vi "Main Page.vi"(8 "error in":errorcluster, 11 "Node Ptr":T1 format="%.0x") -> (0 "error out":errorcluster)   [LabVIEW 2017, in "Waveform-Processing-Custom-Device System Explorer.lvlib"]
uses:
  Waveform-Processing-Custom-Device System Explorer.lvlib
  <vilib>/NI Veristand/Custom Device API/Custom Device Item Ref.ctl
  Shared/Custom Device Settings.ctl
  Shared/Types/FG Action.ctl
  Types/UI Refs Ctl.ctl
  <vilib>/NI Veristand/Custom Device API/Custom Device API.lvlib
  Shared/Single Point/SinglePoint.lvlib
  Shared/Running Average/Running Average.lvlib
  Shared/Waveform-Processing-Custom-Device Shared.lvlib
  Shared/Min Single Point/Min_SP.lvlib
  Shared/Max Single Point/Max_SP.lvlib
panel:
  in  "RMS":bool
  in  "Max":bool
  in  "Min":bool
  out "Number of Channels":u32 caption="# Ch's"
  in  "Refresh Waveform List":bool
  out "Revision":string
  in  "Header 2":cluster{"Section Name":string}={"Section Name"="Custom Device Item Settings"}
  out "Task Rate":dbl caption="Hz"
  in  "Buffer Length":dbl=1.0 caption="Sec" min=1.0 format="%#_6f"
  out "Buffer Length":u32 caption="Samples"
  in  "Description":string
  in  "Remove Channel":bool
  in  "Add Channel":bool
  in  "Selected Waveforms":i32[](listbox)
  in  "Waveform Task":u16(ring) items=["Waveform1"=11, "Waveform2"=15]
  in  "Available Waveforms":i32[](listbox)
  in  "Single-point":bool
  in  "Header":cluster{"Section Name":string}={"Section Name"="Custom Device Item Settings"}
  in  "Name":string
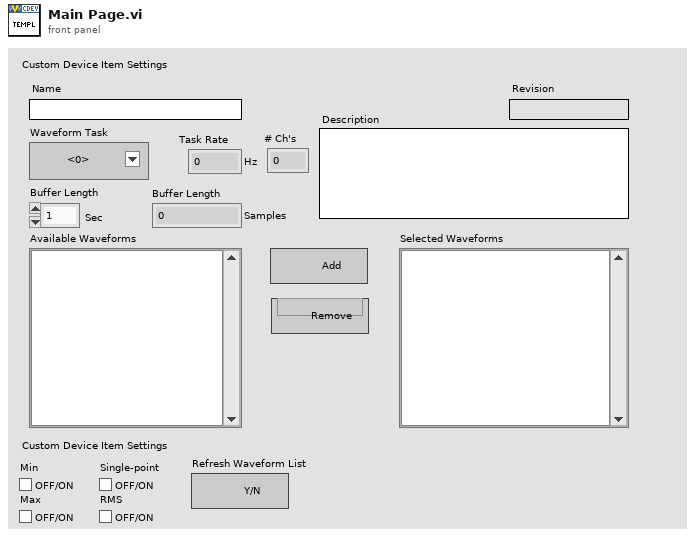
[diagram p1: front panel]
types:
  T1 = typedef "Custom Device API.lvlib/Custom Device Item Ref.ctl" = u64
  T2 = typedef "Waveform-Processing-Custom-Device Shared.lvlib/Custom Device Settings.ctl" = cluster{"CD Task Dependency":T1, "CD Task Dependency Ref":T1, "CD Task Available Wfms":string[], "CD Task Selected Wfms":string[], "Buffer Length (samples)":u32, "Min Enabled":bool, "Max Enabled ":bool, "SP Enabled":bool, "RMS Enabled":bool, "Buffer Length (s)":dbl, "Task Rate":dbl, "Number of DAQ Chanels":u32}
  T3 = typedef "Waveform-Processing-Custom-Device Shared.lvlib/UI Refs Ctl.ctl" = cluster{"Waveform Task":refnum<vi>, "Selected Waveforms":refnum<vi>, "Available Waveforms":refnum<vi>, "Number of Channels":refnum<vi>, "Wfm Task Rate (Hz)":refnum<vi>, "Buffer Length (s)":refnum<vi>, "Buffer Length (samples)":refnum<vi>, "Add Channel":refnum<vi>, "Remove Channel":refnum<vi>, "Min":refnum<vi>, "Max":refnum<vi>, "SP":refnum<vi>, "RMS":refnum<vi>}
  T4 = typedef "Waveform-Processing-Custom-Device Shared.lvlib/FG Action.ctl" = enum8{"GET", "SET"}
  T5 = typedef "Custom Device API.lvlib/Custom Device Item Info.ctl" = cluster{"Name":string, "Is Channel":bool, "GUID":string, "Is Waveform":bool}
  T6 = enum8{"Enabled", "Disabled", "Disabled and Grayed Out"}
  T7 = typedef "Custom Device API.lvlib/Custom Device Commands.ctl" = enum16{"Default", "Item renamed", "Shutdown", "Dynamic button pressed"}
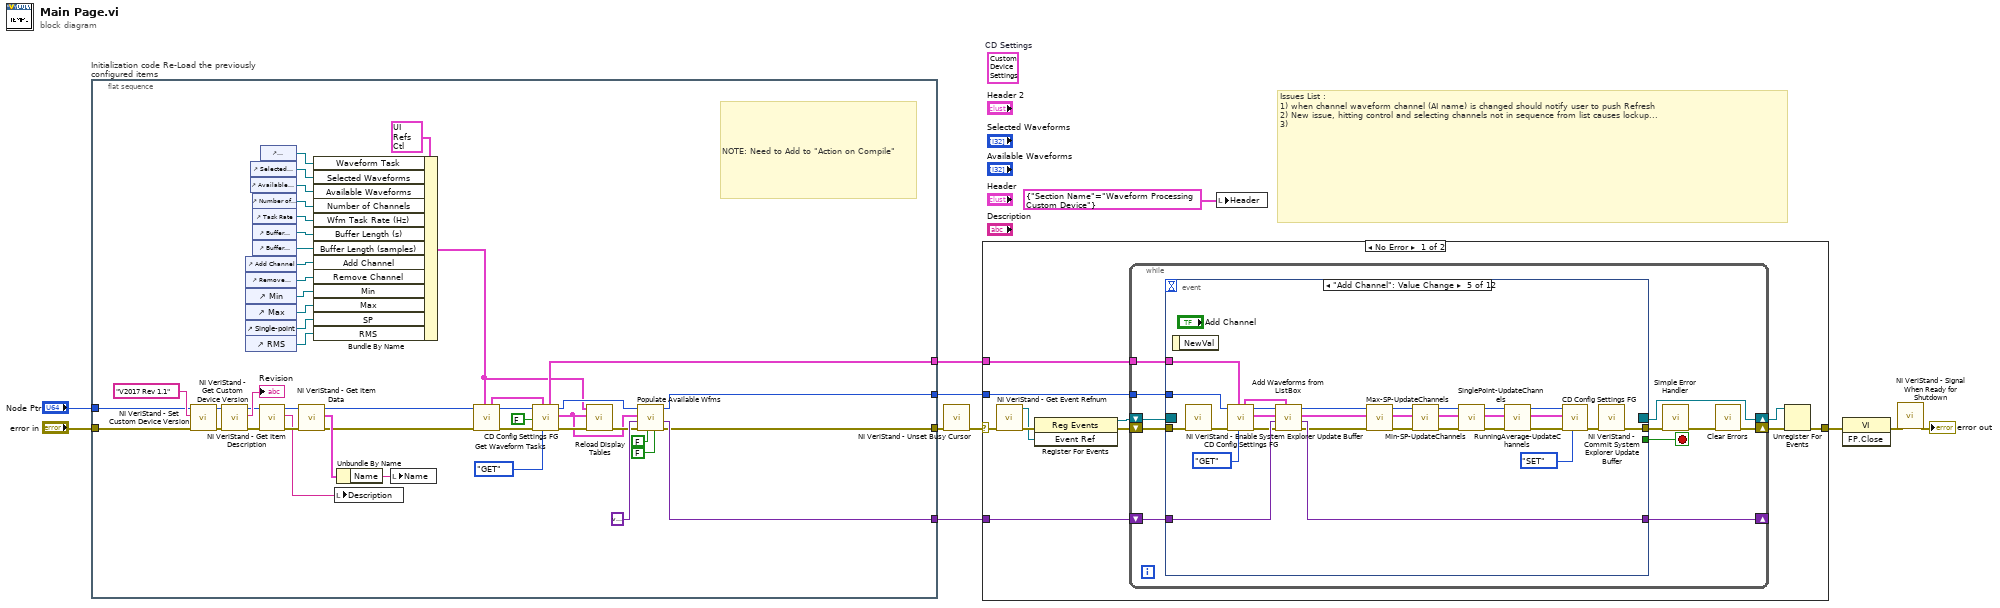
[diagram p0: block diagram]
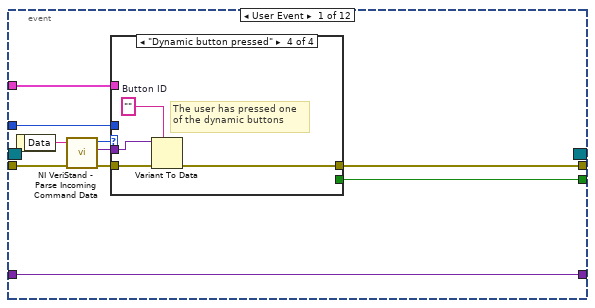
[diagram p2: hidden frame]
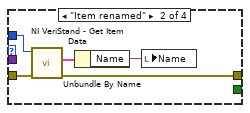
[diagram p4: hidden frame]
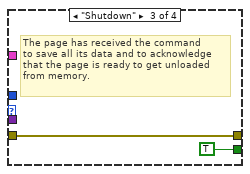
[diagram p5: hidden frame]
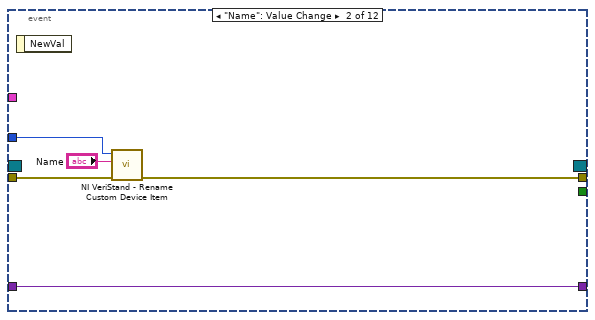
[diagram p6: hidden frame]
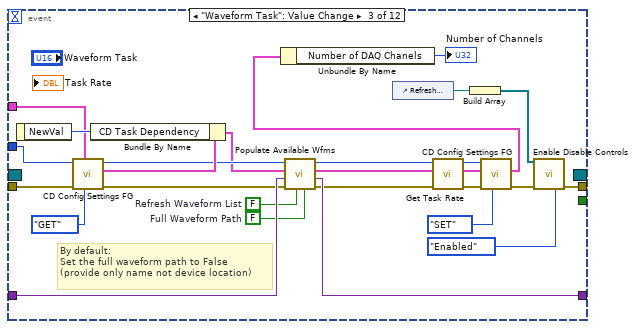
[diagram p7: hidden frame]
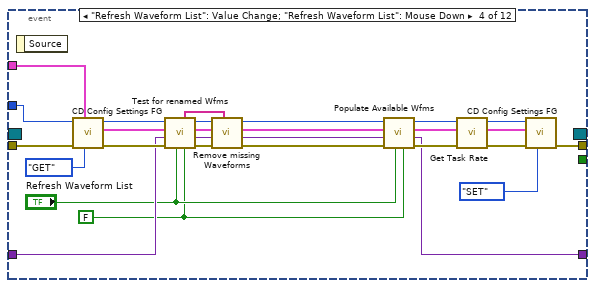
[diagram p8: hidden frame]
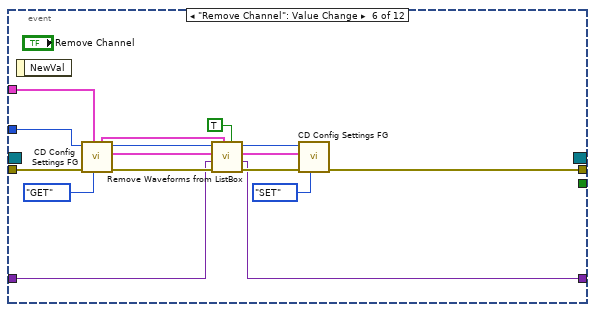
[diagram p9: hidden frame]
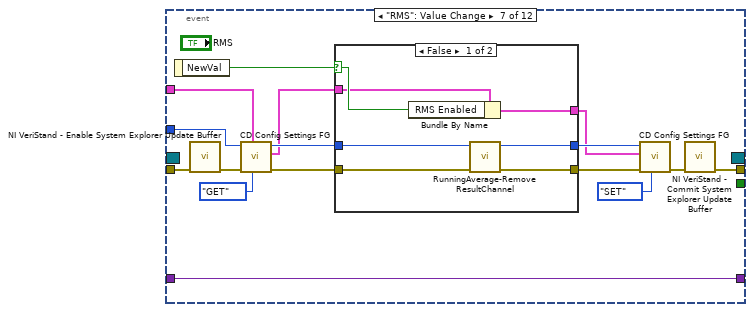
[diagram p10: hidden frame]
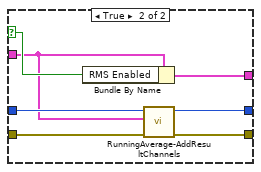
[diagram p11: hidden frame]
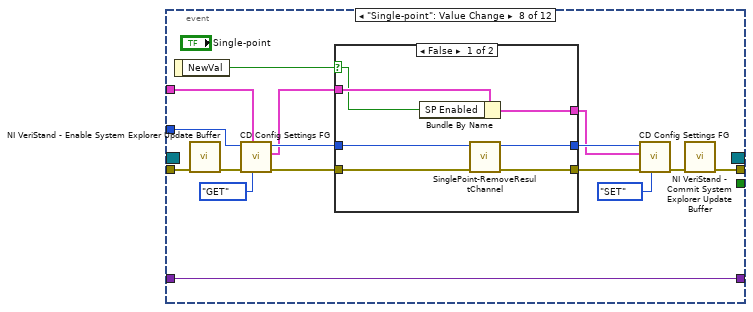
[diagram p12: hidden frame]
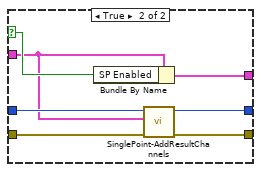
[diagram p13: hidden frame]
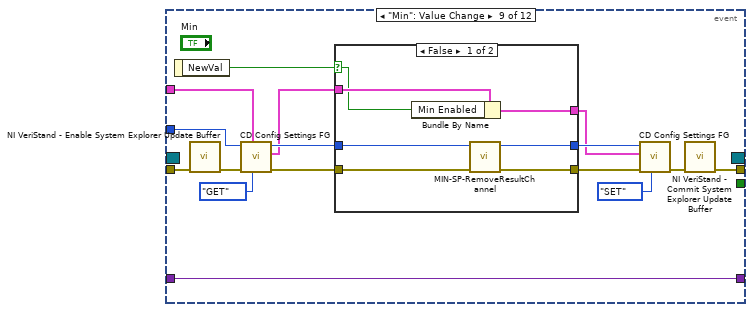
[diagram p14: hidden frame]
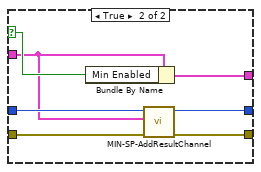
[diagram p15: hidden frame]
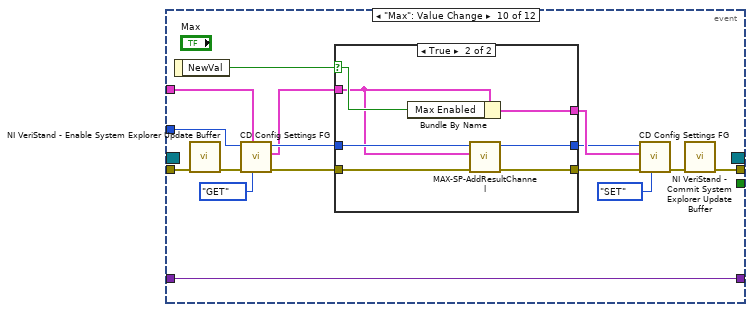
[diagram p16: hidden frame]
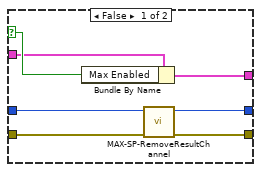
[diagram p17: hidden frame]
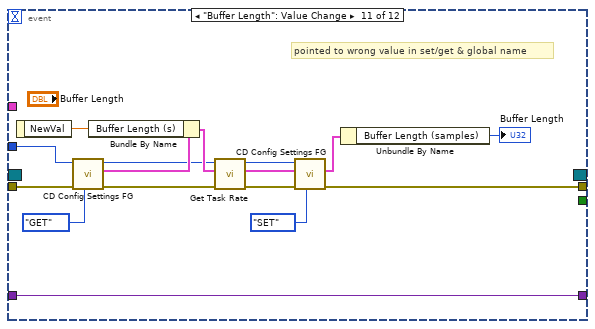
[diagram p18: hidden frame]
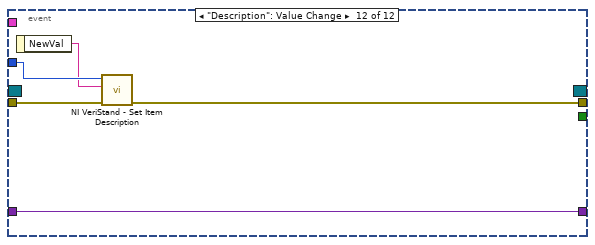
[diagram p19: hidden frame]
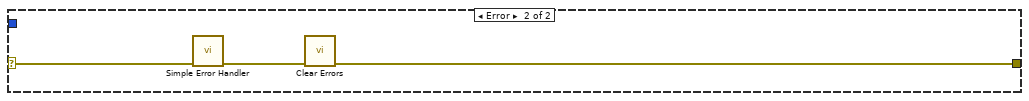
[diagram p20: hidden frame]
diagram:
  (unwired) T2 {"CD Task Dependency"=18446744073709551615, "CD Task Dependency Ref"=18446744073709551615, "CD Task Available Wfms"=[], "CD Task Selected Wfms"=[], "Buffer Length (samples)"=0, "Min Enabled"=FALSE, "Max Enabled "=FALSE, "SP Enabled"=FALSE, "RMS Enabled"=FALSE, "Buffer Length (s)"=0.0, "Task Rate"=0.0, "Number of DAQ Chanels"=0}  # CD Settings
  # "Issues List : \n1) when channel waveform channel (AI name) is changed should notify user to push Refresh\n2) New issue, hitting control and selecting channels not in sequence from list causes lockup...\n3)"
  n1 = flat-sequence "Initialization code Re-Load the previously configured items" {
    tunnel: [w51] -> w4
    tunnel: [w35] -> w7
    tunnel: [w47] -> w6
    tunnel: [w17] -> w5
    tunnel: "error in" -> [w30]
    tunnel: "Node Ptr" -> [w40]
    frame #0 {
      # "NOTE: Need to Add to \"Action on Compile\""
      n2 = call <vilib>:"NI VeriStand - Set Custom Device Version.vi"("error in (no error)"=w30, "Value"="V2017 Rev 1.1", "Device Ref in"=w40) -> ("error out"=w44:errorcluster, "Device Ref out"=w45:T1)  [unwired: 7 in]
      n3 = call <vilib>:"NI VeriStand - Get Custom Device Version.vi"("error in (no error)"=w44, "Device Ref in"=w45) -> ("error out"=w42:errorcluster, "Value"=→"Revision":string, "Device Ref out"=w41:T1)  [unwired: 7 in]
      n4 = control-ref of="Add Channel"() -> (w23:refnum<vi>)
      n5 = control-ref of="Remove Channel"() -> (w22:refnum<vi>)
      n6 = control-ref of="Min"() -> (w13:refnum<vi>)
      n7 = control-ref of="Max"() -> (w21:refnum<vi>)
      n8 = control-ref of="Single-point"() -> (w20:refnum<vi>)
      n9 = control-ref of="RMS"() -> (w19:refnum<vi>)
      n10 = control-ref of="Selected Waveforms"() -> (w28:refnum<vi>)
      n11 = control-ref of="Available Waveforms"() -> (w27:refnum<vi>)
      n12 = control-ref of="Number of Channels"() -> (w26:refnum<vi>)
      n13 = control-ref of="Task Rate"() -> (w25:refnum<vi>)
      n14 = control-ref of="Buffer Length"() -> (w24:refnum<vi>)
      n15 = control-ref of="Buffer Length"() -> (w18:refnum<vi>)
      n16 = call <vilib>:"NI VeriStand - Get Item Description.vi"("error in (no error)"=w42, "Item Ref in"=w41) -> ("error out"=w56:errorcluster, "Description"=w53:string, "Item Ref out"=w57:T1)  [unwired: 7 out]
      n17 = control-ref of="Waveform Task"() -> (w29:refnum<vi>)
      n18 = call <vilib>:"NI VeriStand - Get Item Data.vi"("error in (no error)"=w56, "Item Ref in"=w57) -> ("error out"=w36:errorcluster, "Item Info"=w55:T5, "Item Ref out"=w14:T1)  [unwired: 7 out]
      n19 = Bundle By Name(cluster=T3 {"Waveform Task"=refnum, "Selected Waveforms"=refnum, "Available Waveforms"=refnum, "Number of Channels"=refnum, "Wfm Task Rate (Hz)"=refnum, "Buffer Length (s)"=refnum, "Buffer Length (samples)"=refnum, "Add Channel"=refnum, "Remove Channel"=refnum, "Min"=refnum, "Max"=refnum, "SP"=refnum, "RMS"=refnum} ("UI Refs"), "Waveform Task"=w29, "Selected Waveforms"=w28, "Available Waveforms"=w27, "Number of Channels"=w26, "Wfm Task Rate (Hz)"=w25, "Buffer Length (s)"=w24, "Buffer Length (samples)"=w18, "Add Channel"=w23, "Remove Channel"=w22, "Min"=w13, "Max"=w21, "SP"=w20, "RMS"=w19) -> (w16:T3)
      n20 = local write "Description"(w53) -> ()
      n21 = Unbundle By Name(w55) -> ("Name"=w54:string)
      n22 = local write "Name"(w54) -> ()
      n23 = call "Get Waveform Tasks.vi"("Custom Device ref in"=w14, "error in"=w36, "UI Refs in"=w16) -> ("UI Refs out"=w15:T3, "Custom Device ref out"=w48:T1, "error out"=w34:errorcluster)  [unwired: 5 in]
      n24 = call "CD Config Settings FG.vi"("Action"=FG_Action."GET", "UI Refs"=w15, "Error In"=w34, "Force"=FALSE, "Item Ref"=w48) -> ("Error Out"=w33:errorcluster, "CD Settings out"=w12:T2, "Item Ref out"=w39:T1, "UI Refs out"=w17:T3)  [unwired: 3 in]
      n25 = call "Reload Display Tables.vi"("Error In"=w33, "CD Settings In"=w12, "UI Refs In"=w16) -> ("Error Out"=w32:errorcluster)  [unwired: 8 in]
      n26 = call "Populate Available Wfms.vi"("Full Path info"=FALSE, "Refresh List"=FALSE, "Error In"=w32, "ListBox Variant"=variant, "CD Settings"=w12, "CustomDevice Ref"=w39) -> ("Error Out"=w35:errorcluster, "ListBox Variant"=w51:variant, "CustomDevice Ref"=w47:T1)  [unwired: 1 in, 2 out]
    }
  }
  n27 = call <vilib>:"NI VeriStand - Unset Busy Cursor.vi"("error in (no error)"=w7) -> ("error out"=w8:errorcluster)  [unwired: 10 out]
  n28 = case shown="No Error" w8 {
    selector: w8 -> [w61 w350]
    tunnel: [w65 w348] -> w11
    tunnel: w6 -> [w60 _]
    tunnel: w4 -> [w59 _]
    tunnel: w5 -> [w58 _]
    frame No Error {
      n29 = call <vilib>:"NI VeriStand - Get Event Refnum.vi"("error in (no error)"=w61) -> ("error out"=w68:errorcluster, "Event Ref"=w64:refnum<user-event>)  [unwired: 9 out]
      n30 = register-events(error in=w68, w64) -> (reference out=w62:refnum<event-registration>, error out=w63:errorcluster)  [unwired: 1 in]
      n31 = while {
        shift-right: [w75] -> w66
        shift-left: w63 -> [w72]
        shift-right: [w79] -> w67
        shift-left: w62 -> [w78]
        tunnel: w60 -> [w74]
        shift-right: [w70] -> _
        shift-left: w59 -> [w73]
        tunnel: w58 -> [w69]
        stop <- w77 stop-if-true
        n32 = event shown="[4] \"Add Channel\": Value Change" {
          selector: w78 -> [_ _ _ _ _ _ _ _ _ _ _ _]
          dyn-events: [_ _ _ _ _ _ _ _ _ _ _ _] -> w79
          timeout: _ -> [_ _ _ _ _ _ _ _ _ _ _ _]
          tunnel: w72 -> [w89 w106 w118 w161 w178 w203 w212 w238 w269 w299 w341 w347]
          tunnel: [w85 _ _ _ _ _ _ _ _ _ _ _] -> w77
          tunnel: [w84 w105 w116 w151 w174 w195 w207 w240 w271 w300 w331 w346] -> w71
          tunnel: w74 -> [w82 w103 w130 w160 w190 w206 w218 w247 w276 w310 w330 w345]
          tunnel: [w81 w102 w133 w137 w182 w192 w221 w251 w282 w312 w342 w343] -> w70
          tunnel: w73 -> [w81 w102 w132 w148 w185 w194 w221 w251 w282 w312 w342 w343]
          tunnel: w69 -> [w80 _ w121 w134 w181 w193 w215 w248 w274 w311 _ _]
          event User Event {
            n33 = event-data() -> ("Data"=w88:string)  [unwired: 1 out]
            n34 = call <vilib>:"NI VeriStand - Parse Incoming Command Data.vi"("error in (no error)"=w89, "Incoming data"=w88) -> ("error out"=w87:errorcluster, "Outgoing data"=w83:variant, "Action"=w86:T7)  [unwired: 7 out]
            n35 = case shown="\"Dynamic button pressed\"" w86 {
              tunnel: w87 -> [w90 w95 w96 w101]
              tunnel: [_ _ TRUE _] -> w85
              tunnel: [w90 w93 w96 w98] -> w84
              tunnel: w83 -> [_ _ _ w100]
              tunnel: w82 -> [_ w91 _ _]
              tunnel: w80 -> [_ _ _ _]
              frame "Default", Default {
              }
              frame "Item renamed" {
                n36 = call <vilib>:"NI VeriStand - Get Item Data.vi"("error in (no error)"=w95, "Item Ref in"=w91) -> ("error out"=w93:errorcluster, "Item Info"=w94:T5)  [unwired: 8 out]
                n37 = Unbundle By Name(w94) -> ("Name"=w92:string)
                n38 = local write "Name"(w92) -> ()
              }
              frame "Shutdown" {
                # "The page has received the command \nto save all its data and to acknowledge \nthat the page is ready to get unloaded \nfrom memory."
              }
              frame "Dynamic button pressed" {
                w99 = ""  # Button ID
                # "The user has pressed one \nof the dynamic buttons"
                n39 = Variant To Data(error in=w101, type=w99, Variant=w100) -> (error out=w98:errorcluster)  [unwired: 1 out]
              }
            }
          }
          event "Name": Value Change {
            n40 = event-data() -> ()  [unwired: 2 out]
            n41 = call <vilib>:"NI VeriStand - Rename Custom Device Item.vi"("error in (no error)"=w106, "New Name"="Name", "Item Ref in"=w103) -> ("error out"=w105:errorcluster)  [unwired: 1 in, 7 out]
          }
          event "Waveform Task": Value Change {
            w119 = FALSE  # Full Waveform Path
            w120 = FALSE  # Refresh Waveform List
            # "By default:\nSet the full waveform path to False \n(provide only name not device location)"
            n42 = event-data() -> ("NewVal"=w131:u16)  [unwired: 1 out]
            n43 = call "CD Config Settings FG.vi"("Action"=FG_Action."GET", "UI Refs"=w121, "Error In"=w118, "Item Ref"=w130) -> ("Error Out"=w126:errorcluster, "CD Settings out"=w129:T2, "Item Ref out"=w125:T1)  [unwired: 4 in, 1 out]
            n44 = Bundle By Name(cluster=w129, "CD Task Dependency"=w131) -> (w124:T2)
            n45 = call "Populate Available Wfms.vi"("Full Path info"=w119, "Refresh List"=w120, "Error In"=w126, "ListBox Variant"=w132, "CD Settings"=w124, "CustomDevice Ref"=w125) -> ("Error Out"=w112:errorcluster, "ListBox Variant"=w133:variant, "CD Settings out"=w110:T2, "CustomDevice Ref"=w111:T1)  [unwired: 1 in, 1 out]
            n46 = control-ref of="Refresh Waveform List"() -> (w114:refnum<vi>)
            n47 = call "Get Task Rate.vi"("error in"=w112, "CD Settings"=w110, "CustomDevice Ref"=w111) -> ("error out"=w122:errorcluster, "CD Settings out"=w109:T2, "CustomDevice Ref out"=w123:T1)  [unwired: 6 in]
            n48 = Build Array(w114) -> (w113:refnum<vi>[])
            n49 = call "CD Config Settings FG.vi"("Action"=FG_Action."SET", "Error In"=w122, "CD Settings in"=w109, "Item Ref"=w123) -> ("Error Out"=w117:errorcluster, "CD Settings out"=w108:T2)  [unwired: 4 in, 2 out]
            n50 = Unbundle By Name(w108) -> ("Number of DAQ Chanels"=→"Number of Channels":u32)
            n51 = call "Enable Disable Controls.vi"("Control Group 1"=w113, "Error In"=w117, "Control Group 1 Mode"=T6."Enabled" ("Disabled")) -> ("Error Out"=w116:errorcluster)  [unwired: 12 in]
          }
          event "Refresh Waveform List": Value Change; "Refresh Waveform List": Mouse Down {
            w135 = FALSE ("Full Waveform Path")
            n52 = event-data() -> ()  [unwired: 2 out]
            n53 = call "CD Config Settings FG.vi"("Action"=FG_Action."GET", "UI Refs"=w134, "Error In"=w161, "Item Ref"=w160) -> ("Error Out"=w150:errorcluster, "CD Settings out"=w147:T2, "Item Ref out"=w149:T1)  [unwired: 4 in, 1 out]
            n54 = call "Test for renamed Wfms.vi"("Full Path info"=w135, "Refresh List"="Refresh Waveform List", "Error In"=w150, "ListBox Variant"=w148, "CD Settings"=w147, "CustomDevice Ref"=w149) -> ("Error Out"=w142:errorcluster, "ListBox Variant"=w144:variant, "CD Settings out"=w139:T2, "CustomDevice Ref"=w145:T1, "Names to Remove"=w140:string[])  [unwired: 1 in]
            n55 = call "Remove missing Waveforms.vi"("Names to Remove"=w140, "Error In"=w142, "ListBox Variant In"=w144, "CD Settings in"=w139, "Item Ref In"=w145) -> ("Error Out"=w141:errorcluster, "ListBox Variant Out"=w143:variant, "CD Settings out"=w138:T2, "Item Ref Out"=w146:T1)  [unwired: 3 in]
            n56 = call "Populate Available Wfms.vi"("Full Path info"=w135, "Refresh List"="Refresh Waveform List", "Error In"=w141, "ListBox Variant"=w143, "CD Settings"=w138, "CustomDevice Ref"=w146) -> ("Error Out"=w157:errorcluster, "ListBox Variant"=w137:variant, "CD Settings out"=w156:T2, "CustomDevice Ref"=w155:T1)  [unwired: 1 in, 1 out]
            n57 = call "Get Task Rate.vi"("error in"=w157, "CD Settings"=w156, "CustomDevice Ref"=w155) -> ("error out"=w153:errorcluster, "CD Settings out"=w152:T2, "CustomDevice Ref out"=w154:T1)  [unwired: 6 in]
            n58 = call "CD Config Settings FG.vi"("Action"=FG_Action."SET", "Error In"=w153, "CD Settings in"=w152, "Item Ref"=w154) -> ("Error Out"=w151:errorcluster)  [unwired: 4 in, 3 out]
          }
          event "Add Channel": Value Change {
            n59 = event-data() -> ()  [unwired: 2 out]
            n60 = call <vilib>:"NI VeriStand - Enable System Explorer Update Buffer.vi"("error in (no error)"=w178) -> ("error out"=w177:errorcluster)  [unwired: 10 in]
            n61 = call "CD Config Settings FG.vi"("Action"=FG_Action."GET", "UI Refs"=w181, "Error In"=w177, "Item Ref"=w190) -> ("Error Out"=w184:errorcluster, "CD Settings out"=w187:T2, "Item Ref out"=w186:T1, "UI Refs out"=w183:T3)  [unwired: 4 in]
            n62 = call "Add Waveforms from ListBox.vi"("UI Refs"=w183, "error in"=w184, "Wfm Ref LUT"=w185, "CD Settings in"=w187, "Custom Device Ref in"=w186) -> ("error out"=w176:errorcluster, "Wfm Ref LUT out"=w182:variant, "CD Settings out"=w179:T2, "Custom Device Ref out"=w180:T1)  [unwired: 3 in]
            n63 = call "Max-SP-UpdateChannels.vi"("Error In"=w176, "CD Settings In"=w179, "Item Ref in"=w180) -> ("Error Out"=w172:errorcluster, "CD Settings Out"=w171:T2, "Item Ref Out"=w173:T1)  [unwired: 6 in]
            n64 = call "Min-SP-UpdateChannels.vi"("Error In"=w172, "CD Settings In"=w171, "Item Ref in"=w173) -> ("Error Out"=w168:errorcluster, "CD Settings Out"=w169:T2, "Item Ref Out"=w170:T1)  [unwired: 6 in]
            n65 = call "SinglePoint-UpdateChannels.vi"("Error in"=w168, "CD Settings In"=w169, "Custom Device ref in"=w170) -> ("Error out"=w163:errorcluster, "CD Settings Out"=w165:T2, "Custom Device ref out"=w167:T1)  [unwired: 6 in]
            n66 = call "RunningAverage-UpdateChannels.vi"("Error in"=w163, "CD Settings In"=w165, "Custom Device ref in"=w167) -> ("Error out"=w162:errorcluster, "CD Settings"=w164:T2, "Custom Device ref out"=w166:T1)  [unwired: 6 in]
            n67 = call "CD Config Settings FG.vi"("Action"=FG_Action."SET", "Error In"=w162, "CD Settings in"=w164, "Item Ref"=w166) -> ("Error Out"=w175:errorcluster)  [unwired: 4 in, 3 out]
            n68 = call <vilib>:"NI VeriStand - Commit System Explorer Update Buffer.vi"("error in (no error)"=w175) -> ("error out"=w174:errorcluster)  [unwired: 10 in]
          }
          event "Remove Channel": Value Change {
            n69 = event-data() -> ()  [unwired: 2 out]
            n70 = call "CD Config Settings FG.vi"("Action"=FG_Action."GET", "UI Refs"=w193, "Error In"=w203, "Item Ref"=w206) -> ("Error Out"=w202:errorcluster, "CD Settings out"=w200:T2, "Item Ref out"=w199:T1, "UI Refs out"=w198:T3)  [unwired: 4 in]
            n71 = call "Remove Waveforms from ListBox.vi"("Names List"=TRUE, "UI Refs"=w198, "error in"=w202, "Waveform Ref LUT"=w194, "CD Settings in"=w200, "Custom Device Ref in"=w199) -> ("error out"=w201:errorcluster, "Waveform Ref LUT out"=w192:variant, "CD Settings out"=w196:T2, "Custom Device Ref out"=w197:T1)  [unwired: 2 in]
            n72 = call "CD Config Settings FG.vi"("Action"=FG_Action."SET", "Error In"=w201, "CD Settings in"=w196, "Item Ref"=w197) -> ("Error Out"=w195:errorcluster)  [unwired: 4 in, 3 out]
          }
          event "RMS": Value Change {
            n73 = event-data() -> ("NewVal"=w222:bool)  [unwired: 1 out]
            n74 = call <vilib>:"NI VeriStand - Enable System Explorer Update Buffer.vi"("error in (no error)"=w212) -> ("error out"=w211:errorcluster)  [unwired: 10 in]
            n75 = call "CD Config Settings FG.vi"("Action"=FG_Action."GET", "UI Refs"=w215, "Error In"=w211, "Item Ref"=w218) -> ("Error Out"=w210:errorcluster, "CD Settings out"=w214:T2, "Item Ref out"=w217:T1)  [unwired: 4 in, 1 out]
            n76 = case shown="False" w222 {
              selector: w222 -> [w225 w231]
              tunnel: w210 -> [w229 w234]
              tunnel: [w227 w235] -> w209
              tunnel: w217 -> [w228 w236]
              tunnel: [w224 w233] -> w216
              tunnel: w214 -> [w223 w230]
              tunnel: [w226 w232] -> w213
              frame False {
                n77 = Bundle By Name(cluster=w223, "RMS Enabled"=w225) -> (w226:T2)
                n78 = call "RunningAverage-RemoveResultChannel.vi"("Error in"=w229, "Custom Device ref"=w228) -> ("Error out"=w227:errorcluster, "Custom Device ref out"=w224:T1)  [unwired: 8 in]
              }
              frame True {
                n79 = Bundle By Name(cluster=w230, "RMS Enabled"=w231) -> (w232:T2)
                n80 = call "RunningAverage-AddResultChannels.vi"("Error in"=w234, "CD Settings in"=w230, "Custom Device ref"=w236) -> ("Error out"=w235:errorcluster, "Custom Device ref out"=w233:T1)  [unwired: 7 in]
              }
            }
            n81 = call "CD Config Settings FG.vi"("Action"=FG_Action."SET", "Error In"=w209, "CD Settings in"=w213, "Item Ref"=w216) -> ("Error Out"=w208:errorcluster)  [unwired: 4 in, 3 out]
            n82 = call <vilib>:"NI VeriStand - Commit System Explorer Update Buffer.vi"("error in (no error)"=w208) -> ("error out"=w207:errorcluster)  [unwired: 10 in]
          }
          event "Single-point": Value Change {
            n83 = event-data() -> ("NewVal"=w252:bool)  [unwired: 1 out]
            n84 = call <vilib>:"NI VeriStand - Enable System Explorer Update Buffer.vi"("error in (no error)"=w238) -> ("error out"=w237:errorcluster)  [unwired: 10 in]
            n85 = call "CD Config Settings FG.vi"("Action"=FG_Action."GET", "UI Refs"=w248, "Error In"=w237, "Item Ref"=w247) -> ("Error Out"=w239:errorcluster, "CD Settings out"=w244:T2, "Item Ref out"=w246:T1)  [unwired: 4 in, 1 out]
            n86 = case shown="False" w252 {
              selector: w252 -> [w253 w261]
              tunnel: w239 -> [w258 w266]
              tunnel: [w257 w265] -> w242
              tunnel: w246 -> [w259 w264]
              tunnel: [w256 w263] -> w245
              tunnel: w244 -> [w255 w260]
              tunnel: [w254 w262] -> w243
              frame False {
                n87 = Bundle By Name(cluster=w255, "SP Enabled"=w253) -> (w254:T2)
                n88 = call "SinglePoint-RemoveResultChannel.vi"("Error in"=w258, "Custom Device ref"=w259) -> ("Error out"=w257:errorcluster, "Custom Device ref out"=w256:T1)  [unwired: 8 in]
              }
              frame True {
                n89 = Bundle By Name(cluster=w260, "SP Enabled"=w261) -> (w262:T2)
                n90 = call "SinglePoint-AddResultChannels.vi"("Error in"=w266, "CD Settings in"=w260, "Custom Device ref"=w264) -> ("Error out"=w265:errorcluster, "Custom Device ref out"=w263:T1)  [unwired: 7 in]
              }
            }
            n91 = call "CD Config Settings FG.vi"("Action"=FG_Action."SET", "Error In"=w242, "CD Settings in"=w243, "Item Ref"=w245) -> ("Error Out"=w241:errorcluster)  [unwired: 4 in, 3 out]
            n92 = call <vilib>:"NI VeriStand - Commit System Explorer Update Buffer.vi"("error in (no error)"=w241) -> ("error out"=w240:errorcluster)  [unwired: 10 in]
          }
          event "Min": Value Change {
            n93 = event-data() -> ("NewVal"=w275:bool)  [unwired: 1 out]
            n94 = call <vilib>:"NI VeriStand - Enable System Explorer Update Buffer.vi"("error in (no error)"=w269) -> ("error out"=w268:errorcluster)  [unwired: 10 in]
            n95 = call "CD Config Settings FG.vi"("Action"=FG_Action."GET", "UI Refs"=w274, "Error In"=w268, "Item Ref"=w276) -> ("Error Out"=w270:errorcluster, "CD Settings out"=w267:T2, "Item Ref out"=w277:T1)  [unwired: 4 in, 1 out]
            n96 = case shown="False" w275 {
              selector: w275 -> [w284 w292]
              tunnel: w270 -> [w283 w291]
              tunnel: [w289 w296] -> w273
              tunnel: w277 -> [w287 w293]
              tunnel: [w288 w295] -> w280
              tunnel: w267 -> [w286 w290]
              tunnel: [w285 w294] -> w278
              frame False {
                n97 = Bundle By Name(cluster=w286, "Min Enabled"=w284) -> (w285:T2)
                n98 = call "MIN-SP-RemoveResultChannel.vi"("Error In"=w283, "Item Ref in"=w287) -> ("Error Out"=w289:errorcluster, "Item Ref out"=w288:T1)  [unwired: 8 in]
              }
              frame True {
                n99 = Bundle By Name(cluster=w290, "Min Enabled"=w292) -> (w294:T2)
                n100 = call "MIN-SP-AddResultChannel.vi"("Error In"=w291, "CD Settings"=w290, "Device Ref in"=w293) -> ("Error Out"=w296:errorcluster, "Device Ref Out"=w295:T1)  [unwired: 7 in]
              }
            }
            n101 = call "CD Config Settings FG.vi"("Action"=FG_Action."SET", "Error In"=w273, "CD Settings in"=w278, "Item Ref"=w280) -> ("Error Out"=w272:errorcluster)  [unwired: 4 in, 3 out]
            n102 = call <vilib>:"NI VeriStand - Commit System Explorer Update Buffer.vi"("error in (no error)"=w272) -> ("error out"=w271:errorcluster)  [unwired: 10 in]
          }
          event "Max": Value Change {
            n103 = event-data() -> ("NewVal"=w304:bool)  [unwired: 1 out]
            n104 = call <vilib>:"NI VeriStand - Enable System Explorer Update Buffer.vi"("error in (no error)"=w299) -> ("error out"=w298:errorcluster)  [unwired: 10 in]
            n105 = call "CD Config Settings FG.vi"("Action"=FG_Action."GET", "UI Refs"=w311, "Error In"=w298, "Item Ref"=w310) -> ("Error Out"=w303:errorcluster, "CD Settings out"=w306:T2, "Item Ref out"=w309:T1)  [unwired: 4 in, 1 out]
            n106 = case shown="True" w304 {
              selector: w304 -> [w315 w321]
              tunnel: w303 -> [w318 w325]
              tunnel: [w319 w326] -> w302
              tunnel: w309 -> [w317 w324]
              tunnel: [w316 w323] -> w297
              tunnel: w306 -> [w314 w320]
              tunnel: [w313 w322] -> w305
              frame False {
                n107 = Bundle By Name(cluster=w314, "Max Enabled"=w315) -> (w313:T2)
                n108 = call "MAX-SP-RemoveResultChannel.vi"("Error In"=w318, "Device Ref in"=w317) -> ("Error Out"=w319:errorcluster, "Device Ref Out"=w316:T1)  [unwired: 8 in]
              }
              frame True {
                n109 = Bundle By Name(cluster=w320, "Max Enabled"=w321) -> (w322:T2)
                n110 = call "MAX-SP-AddResultChannel.vi"("Error In"=w325, "CD Settings in"=w320, "Device Ref in"=w324) -> ("Error Out"=w326:errorcluster, "Device Ref Out"=w323:T1)  [unwired: 7 in]
              }
            }
            n111 = call "CD Config Settings FG.vi"("Action"=FG_Action."SET", "Error In"=w302, "CD Settings in"=w305, "Item Ref"=w297) -> ("Error Out"=w301:errorcluster)  [unwired: 4 in, 3 out]
            n112 = call <vilib>:"NI VeriStand - Commit System Explorer Update Buffer.vi"("error in (no error)"=w301) -> ("error out"=w300:errorcluster)  [unwired: 10 in]
          }
          event "Buffer Length": Value Change {
            # "pointed to wrong value in set/get & global name"
            n113 = event-data() -> ("NewVal"=w338:dbl)  [unwired: 1 out]
            n114 = call "CD Config Settings FG.vi"("Action"=FG_Action."GET", "Error In"=w341, "Item Ref"=w330) -> ("Error Out"=w336:errorcluster, "CD Settings out"=w339:T2, "Item Ref out"=w335:T1)  [unwired: 5 in, 1 out]
            n115 = Bundle By Name(cluster=w339, "Buffer Length (s)"=w338) -> (w337:T2)
            n116 = call "Get Task Rate.vi"("error in"=w336, "CD Settings"=w337, "CustomDevice Ref"=w335) -> ("error out"=w334:errorcluster, "CD Settings out"=w329:T2, "CustomDevice Ref out"=w333:T1)  [unwired: 6 in]
            n117 = call "CD Config Settings FG.vi"("Action"=FG_Action."SET", "Error In"=w334, "CD Settings in"=w329, "Item Ref"=w333) -> ("Error Out"=w331:errorcluster, "CD Settings out"=w328:T2)  [unwired: 4 in, 2 out]
            n118 = Unbundle By Name(w328) -> ("Buffer Length (samples)"=→"Buffer Length":u32)
          }
          event "Description": Value Change {
            n119 = event-data() -> ("NewVal"=w344:string)  [unwired: 1 out]
            n120 = call <vilib>:"NI VeriStand - Set Item Description.vi"("error in (no error)"=w347, "Description"=w344, "Item Ref in"=w345) -> ("error out"=w346:errorcluster)  [unwired: 8 out]
          }
        }
        n121 = call <vilib>:"Simple Error Handler.vi"("error in (no error)"=w71) -> ("error out"=w76:errorcluster)  [unwired: 1 in, 7 out]
        n122 = call <vilib>:"Clear Errors.vi"("error in (no error)"=w76) -> ("error out"=w75:errorcluster)  [unwired: 1 in, 5 out]
      }
      n123 = Unregister For Events(event registration refnum=w67, error in=w66) -> (error out=w65:errorcluster)
    }
    frame Error {
      n124 = call <vilib>:"Simple Error Handler.vi"("error in (no error)"=w350) -> ("error out"=w349:errorcluster)  [unwired: 1 in, 7 out]
      n125 = call <vilib>:"Clear Errors.vi"("error in (no error)"=w349) -> ("error out"=w348:errorcluster)  [unwired: 1 in, 5 out]
    }
  }
  n126 = local write "Header"(cluster{"Section Name":string} {"Section Name"="Waveform Processing Custom Device"} ("Header")) -> ()
  n127 = invoke class="VI" method="FP.Close"(error in=w11) -> (error out=w10:errorcluster)  [unwired: 2 in, 2 out]
  n128 = call <vilib>:"NI VeriStand - Signal When Ready for Shutdown.vi"("error in (no error)"=w10) -> ("error out"=→"error out":errorcluster)  [unwired: 10 out]
